vi "Extract String.vi"(8 "Input String":string, 9 "Text After String":string, 10 "Text Before String":string) -> (3 "Value String":string)   [LabVIEW 2021, in "BS120x Driver.lvlib" / "ENET_BS1200.lvclass"]
uses:
  ENET_BS1200.lvclass
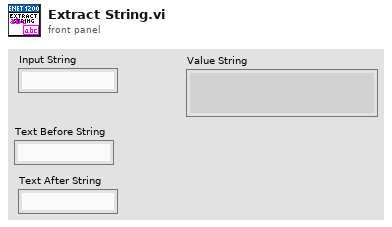
[diagram p1: front panel]
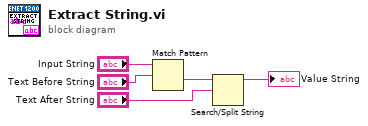
[diagram p0: block diagram]
diagram:
  n1 = Match Pattern(string="Input String", regular expression="Text Before String") -> (after substring=w4:string)  [unwired: 1 in, 3 out]
  n2 = Search/Split String(string=w4, search string/char (-)="Text After String") -> (substring before match=→"Value String":string)  [unwired: 1 in, 2 out]
